vi "Write Channel to Text Log File (U8).vi"(6 "Data":u8[](array[numeric]), 8 "error in (no error)":errorcluster, 9 "Channel Name in":string, 10 "Group Name in":string, 11 "Text Log File in":refnum<class "Text Log File.lvclass">) -> (0 "error out":errorcluster, 3 "Text Log File out":refnum<class "Text Log File.lvclass">)   [LabVIEW 2015, in "Text Log File.lvclass"]
doc: "Writes data to the text file using the specified delimiter and format string. The channel and group names are ignored. The header for the file should be written in advance using Write Log Header.vi."
uses:
  Text Log File.lvclass
  Text Log File.lvclass/Text Log File.ctl
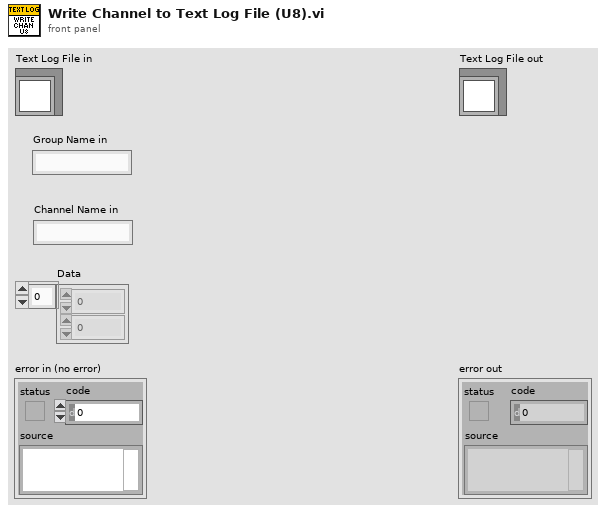
[diagram p1: front panel]
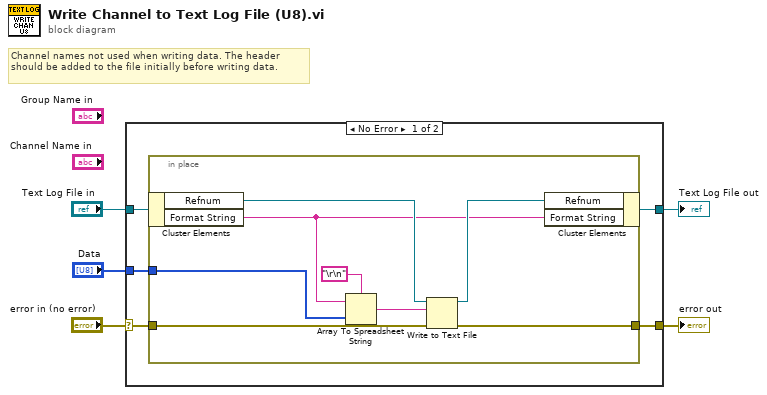
[diagram p0: block diagram]
diagram:
  # "Channel names not used when writing data. The header should be added to the file initially before writing data."
  n1 = case shown="No Error" "error in (no error)" {
    selector: "error in (no error)" -> [w6 w19]
    tunnel: [w10 w20] -> w5
    tunnel: "Data" -> [w9 _]
    tunnel: [w8 w19] -> w3
    tunnel: "Text Log File in" -> [w7 w20]
    frame No Error {
      n2 = in-place {
        in-place-border: w6 -> [w18]
        in-place-border: w9 -> [w12]
        in-place-border: [w16] -> w8
        n3 = in-place-cluster #1(w7) -> ("Refnum"=w15:refnum<file>, "Format String"=w14:string)
        n4 = Array To Spreadsheet String(delimiter (Tab)="\r\n", array=w12, 3:w14) -> (spreadsheet string=w13:string)
        n5 = Write to Text File(file (use dialog)=w15, text=w13, error in=w18) -> (refnum out=w17:refnum<file>, error out=w16:errorcluster)  [unwired: 1 in, 1 out]
        n6 = in-place-cluster #1("Refnum"=w17, "Format String"=w14) -> (w10:refnum<class "Text Log File.lvclass">)
      }
    }
    frame Error {
    }
  }
  "error out" <- w3
  "Text Log File out" <- w5
